vi "Control Dead zone.vi"(10 "dead zone":dbl, 11 "control Value":dbl) -> (3 "output Value":dbl)   [LabVIEW 2020]
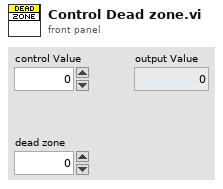
[diagram p1: front panel]
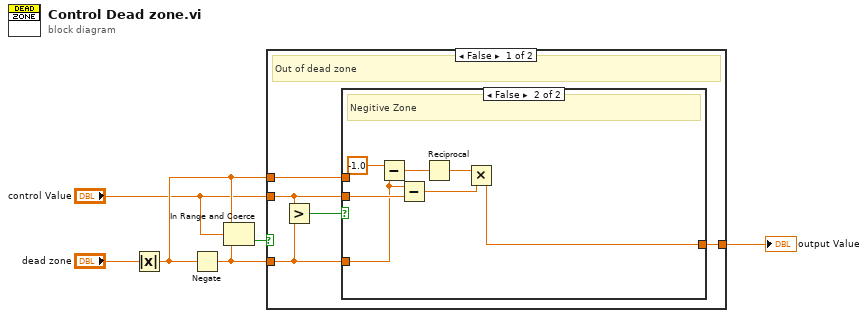
[diagram p0: block diagram]
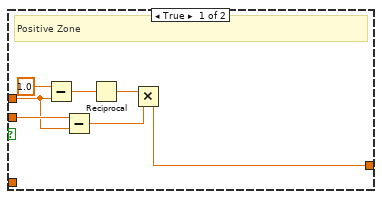
[diagram p2: hidden frame]
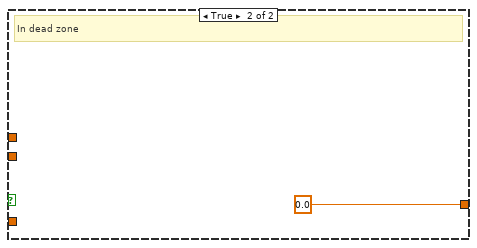
[diagram p3: hidden frame]
diagram:
  n1 = Absolute Value(x="dead zone") -> (abs(x)=w3:dbl)
  n2 = Negate(x=w3) -> (-x=w2:dbl)
  n3 = In Range and Coerce(upper limit=w3, x="control Value", lower limit=w2) -> (In Range?=w5:bool)  [unwired: 1 out]
  n4 = case shown="False" w5 {
    tunnel: "control Value" -> [w10 _]
    tunnel: [w7 0.0] -> w4
    tunnel: w3 -> [w9 _]
    tunnel: w2 -> [w8 _]
    frame False {
      # "Out of dead zone"
      n5 = Greater?(x=w10, y=w8) -> (0:w11:bool)
      n6 = case shown="False" w11 {
        tunnel: w10 -> [w16 w20]
        tunnel: w9 -> [w15 _]
        tunnel: w8 -> [_ w19]
        tunnel: [w12 w21] -> w7
        frame True {
          # "Positive Zone"
          n7 = Subtract(x=1.0, y=w15) -> (x-y=w17:dbl)
          n8 = Subtract(x=w16, y=w15) -> (x-y=w13:dbl)
          n9 = Reciprocal(x=w17) -> (1/x=w14:dbl)
          n10 = Multiply(x=w14, y=w13) -> (x*y=w12:dbl)
        }
        frame False {
          # "Negitive Zone"
          n11 = Subtract(x=-1.0, y=w19) -> (x-y=w24:dbl)
          n12 = Subtract(x=w19, y=w20) -> (x-y=w22:dbl)
          n13 = Reciprocal(x=w24) -> (1/x=w23:dbl)
          n14 = Multiply(x=w23, y=w22) -> (x*y=w21:dbl)
        }
      }
    }
    frame True {
      # "In dead zone"
    }
  }
  "output Value" <- w4
